vi "Get Current Group.vi"(8 "error in (no error)":errorcluster, 11 "Waveform TDMS Log File Specification in":refnum<class "Waveform TDMS Log File Specification.lvclass">) -> (0 "error out":errorcluster, 2 "Current Group":string, 3 "Waveform TDMS Log File Specification out":refnum<class "Waveform TDMS Log File Specification.lvclass">)   [LabVIEW 2015, in "Waveform TDMS Log File Specification.lvclass"]
uses:
  Waveform TDMS Log File Specification.lvclass
  Waveform TDMS Log File Specification.lvclass/Waveform TDMS Log File Specification.ctl
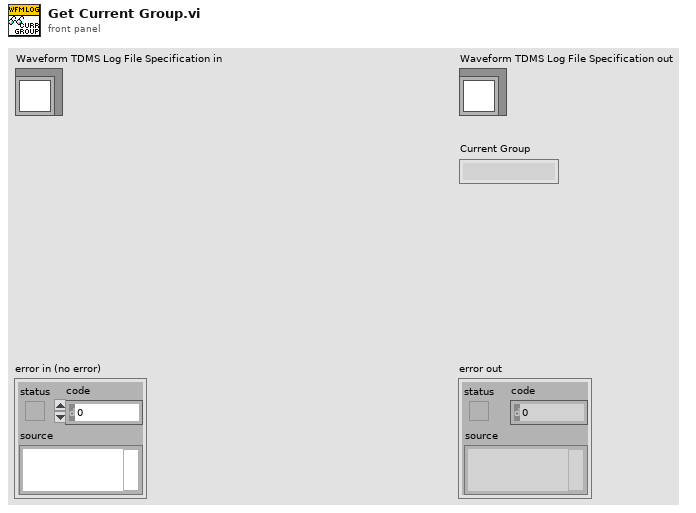
[diagram p1: front panel]
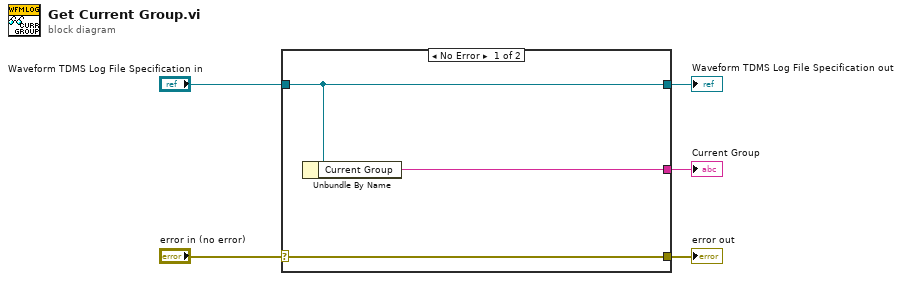
[diagram p0: block diagram]
diagram:
  n1 = case shown="No Error" "error in (no error)" {
    selector: "error in (no error)" -> [w8 w9]
    tunnel: [w8 w9] -> w4
    tunnel: [w7 w10] -> w2
    tunnel: "Waveform TDMS Log File Specification in" -> [w7 w10]
    tunnel: [w6 _] -> w1
    frame No Error {
      n2 = Unbundle By Name(w7) -> ("Current Group"=w6:string)
    }
    frame Error {
    }
  }
  "error out" <- w4
  "Waveform TDMS Log File Specification out" <- w2
  "Current Group" <- w1
